vi "Remove_duplicated_XY_val.vi"(2 "Y values":dbl[](array[numeric]), 3 "Sorted X values":dbl[](array[numeric])) -> (0 "Y Out":dbl[](array[numeric]), 1 "X out":dbl[](array[numeric]))   [LabVIEW 2011]
panel:
  out "No of Unique values":i32
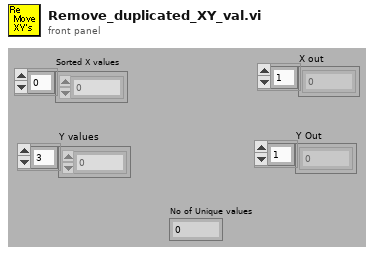
[diagram p1: front panel]
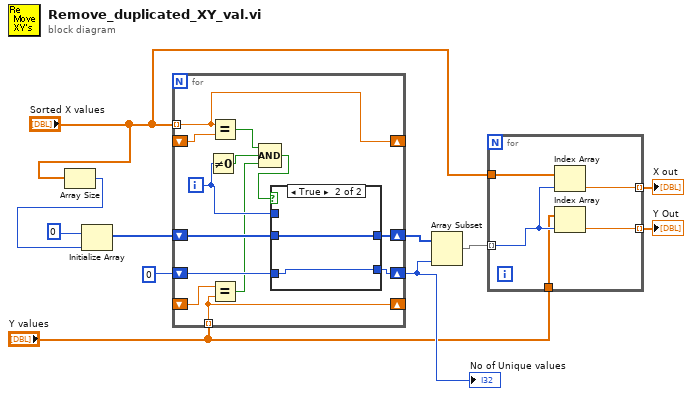
[diagram p0: block diagram]
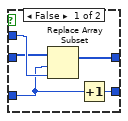
[diagram p2: hidden frame]
diagram:
  n1 = Array Size(array="Sorted X values") -> (size(s)=w10:i32)
  n2 = Initialize Array(0, w10) -> (w9:i32[])
  n3 = for {
    shift-right: [w23] -> _
    shift-left: _ -> [w24]
    tunnel: "Sorted X values" -> [w23] mode=indexing
    shift-right: [w19] -> w7
    shift-left: w9 -> [w21]
    shift-right: [w17] -> w6
    shift-left: 0 -> [w18]
    shift-right: [w16] -> _
    shift-left: _ -> [w15]
    tunnel: "Y values" -> [w16] mode=indexing
    i -> [w20]
    n4 = Not Equal To 0?(x=w20) -> (x != 0?=w13:bool)
    n5 = Equal?(x=w23, y=w24) -> (x = y?=w14:bool)
    n6 = Equal?(x=w15, y=w16) -> (x = y?=w12:bool)
    n7 = Compound Arithmetic op=AND(w14, w13, w12) -> (w22:bool)
    n8 = case shown="True" w22 {
      tunnel: w21 -> [w26 w31]
      tunnel: w20 -> [w29 _]
      tunnel: [w25 w31] -> w19
      tunnel: w18 -> [w28 w30]
      tunnel: [w27 w30] -> w17
      frame False {
        n9 = Replace Array Subset(array=w26, new element=w29, index=w28) -> (w25:i32[])
        n10 = Increment(x=w28) -> (x+1=w27:i32)
      }
      frame True {
      }
    }
  }
  "No of Unique values" <- w6
  n11 = Array Subset(array=w7, length=w6) -> (w5:i32[])  [unwired: 1 in]
  n12 = for {
    tunnel: w5 -> [w36] mode=indexing
    tunnel: "Sorted X values" -> [w35]
    tunnel: "Y values" -> [w34]
    tunnel: [w33] -> w2 mode=indexing
    tunnel: [w32] -> w3 mode=indexing
    n13 = Index Array(array=w35, index=w36) -> (element=w32:dbl)
    n14 = Index Array(array=w34, index=w36) -> (element=w33:dbl)
  }
  "X out" <- w3
  "Y Out" <- w2
